vi "导入预设波形.vi"(11 "导入tdms文件参数":T1) -> (2 "预设波形数组":dbl[][](array[numeric]))   [LabVIEW 2018]
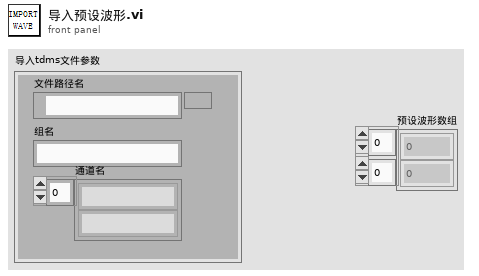
[diagram p1: front panel]
types:
  T1 = cluster{"文件路径名":path, "组名":string, "通道名":string[]}
  T2 = enum16{"open", "open or create", "create or replace", "create", "open (read-only)"}
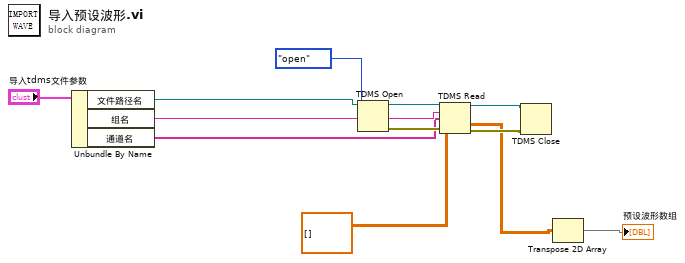
[diagram p0: block diagram]
diagram:
  n1 = Unbundle By Name("导入tdms文件参数") -> ("文件路径名"=w7:path, "组名"=w6:string, "通道名"=w5:string[])
  n2 = TDMS Open(10:T2."open" ("operation (0:open)"), 11:w7) -> (0:w10:errorcluster, 3:w11:refnum<k34>)  [unwired: 5 in]
  n3 = TDMS Read(0:w11, 5:w6, 7:w5, 11:w10, 12:dbl[][] []) -> (4:w4:refnum<k34>, 10:w2:dbl[][], 15:w3:errorcluster)  [unwired: 3 in, 3 out]
  n4 = TDMS Close(8:w3, 11:w4) -> ()  [unwired: 2 out]
  n5 = Transpose 2D Array(2D array=w2) -> (transposed array=→"预设波形数组":dbl[][])
